vi "Write Player.vi"(10 "Player":string, 11 "JoinGame Msg in":refnum<class "JoinGame Msg.lvclass">) -> (3 "JoinGame Msg out":refnum<class "JoinGame Msg.lvclass">)   [LabVIEW 2014, in "GoBang.lvlib" / "JoinGame Msg.lvclass"]
uses:
  JoinGame Msg.lvclass
  JoinGame Msg.lvclass/JoinGame Msg.ctl
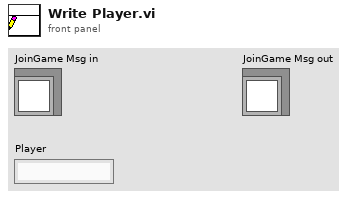
[diagram p1: front panel]
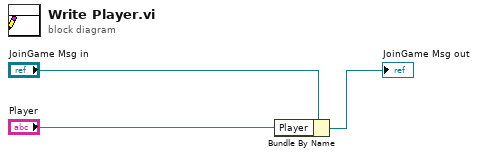
[diagram p0: block diagram]
diagram:
  n1 = Bundle By Name(cluster="JoinGame Msg in", "Player"="Player") -> (→"JoinGame Msg out":refnum<class "JoinGame Msg.lvclass">)
